vi "Player.vi"(8 "error in (no error)":errorcluster, 11 "Player in":refnum<class "Player.lvclass">) -> (0 "error out":errorcluster, 3 "Player out":refnum<class "Player.lvclass">)   [LabVIEW 2017, in "Player.lvclass"]
uses:
  Player.lvclass
  ReadyState Class/ReadyState.lvclass
  C:/Users/fflores/Documents/LabVIEW-Open-Projects/LabIVEW OOP Design Patterns/State Pattern/State Class/State.lvclass
  Player.lvclass/Player.ctl
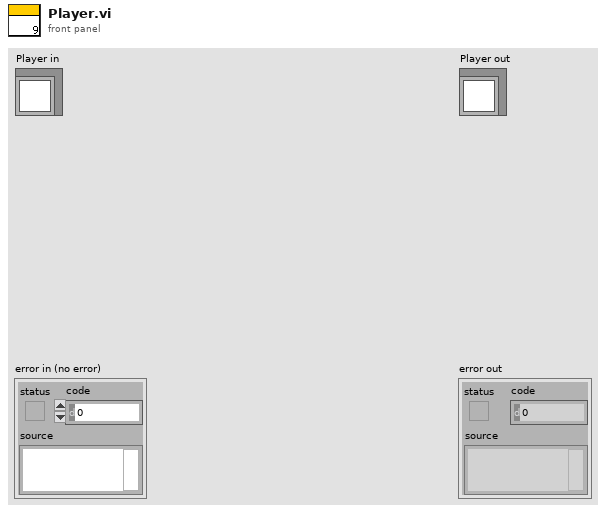
[diagram p1: front panel]
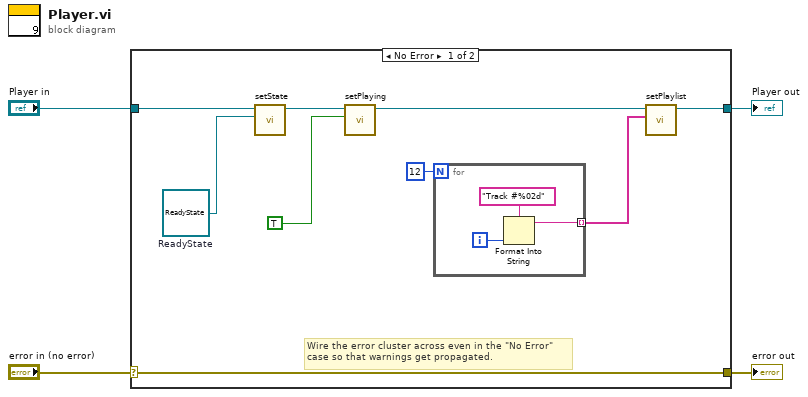
[diagram p0: block diagram]
diagram:
  n1 = case shown="No Error" "error in (no error)" {
    selector: "error in (no error)" -> [w13 w18]
    tunnel: [w13 w18] -> w3
    tunnel: [w6 w17] -> w2
    tunnel: "Player in" -> [w12 w17]
    frame No Error {
      w10 = refnum<class "ReadyState.lvclass"> refnum  # ReadyState
      # "Wire the error cluster across even in the \"No Error\"\ncase so that warnings get propagated."
      n2 = call "setState.vi"("State.lvclass"=w10, "Player in"=w12) -> ("Player out"=w11:refnum<class "Player.lvclass">)  [unwired: 8 in, 1 out]
      n3 = call "setPlaying.vi"("playing"=TRUE, "Player in"=w11) -> ("Player out"=w9:refnum<class "Player.lvclass">)  [unwired: 8 in, 1 out]
      n4 = for {
        N: 12 -> [_]
        tunnel: [w14] -> w5 mode=indexing
        i -> [w15]
        n5 = Format Into String(format string="Track #%02d", w15) -> (resulting string=w14:string)  [unwired: 2 in, 1 out]
      }
      n6 = call "setPlaylist.vi"("Playlist"=w5, "Player in"=w9) -> ("Player out"=w6:refnum<class "Player.lvclass">)  [unwired: 8 in, 1 out]
    }
    frame Error {
    }
  }
  "error out" <- w3
  "Player out" <- w2
